vi "vector_length.vi"(1 "v_y":dbl, 2 "v_x":dbl) -> (0 "||v||":dbl)   [LabVIEW 2020]
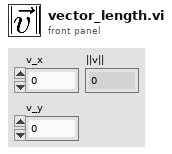
[diagram p1: front panel]
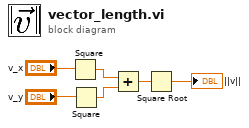
[diagram p0: block diagram]
diagram:
  n1 = Square(x="v_x") -> (x^2=w6:dbl)
  n2 = Square(x="v_y") -> (x^2=w5:dbl)
  n3 = Add(x=w6, y=w5) -> (x+y=w4:dbl)
  n4 = Square Root(x=w4) -> (sqrt(x)=→"||v||":dbl)
